vi "Vaisala_parse_response.vi"(1 "HMP response string":string) -> (4 "Numerics":dbl[](array[numeric]) format="%.2f", 5 "Error":bool, 6 "Error notes":string)   [LabVIEW 2010]
panel:
  # "The correct \"FORM\" command for HMP configuration is:\nRH=\\UUU.UU\\ \\uuu\\ T=\\TTT.TT\\ \\uu\\ Td=\\DDD.DD\\ \\uu\\\\r>"
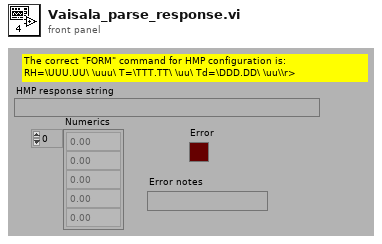
[diagram p1: front panel]
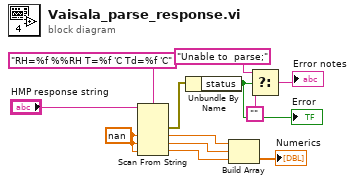
[diagram p0: block diagram]
diagram:
  w1 = nan ("Default Value 1")
  n1 = Scan From String(format string="RH=%f %%RH T=%f 'C Td=%f 'C" ("Format String"), input string="HMP response string", default 1=w1, default 2=w1, default 3=w1) -> (error out=w8:errorcluster, output 1=w10:dbl, output 2=w11:dbl, output 3=w4:dbl)  [unwired: 2 in, 2 out]
  n2 = Unbundle By Name(w8) -> ("status"=w2:bool)
  "Error" <- w2
  n3 = Build Array(w10, w11, w4) -> (→"Numerics":dbl[])
  n4 = Select(t="Unable to  parse;", s=w2, f="") -> (s? t:f=→"Error notes":string)
